vi "3.11-Threshold Lidar Data.vi"(2 "Angle Array":dbl[](array[numeric]), 3 "Magnitude Array":dbl[](array[numeric])) -> (0 "Y (mm)":dbl[](array[numeric]), 1 "X (mm)":dbl[](array[numeric]))   [LabVIEW 2010]
uses:
  3.0-Global.vi
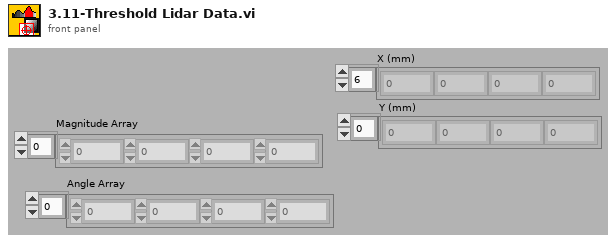
[diagram p1: front panel]
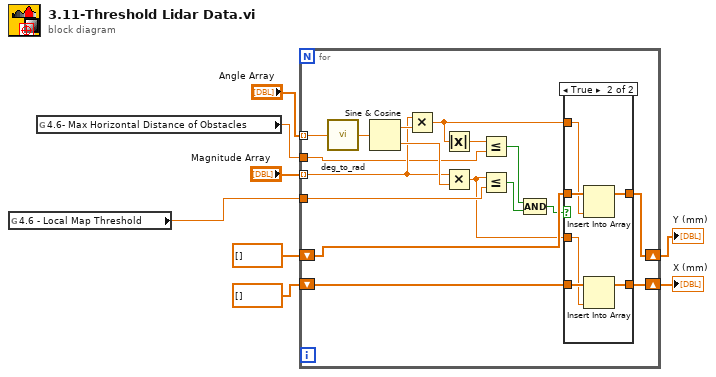
[diagram p0: block diagram]
diagram:
  n1 = global read "3.0-Global.vi" "4.6 - Local Map Threshold"() -> (w1:dbl)
  n2 = global read "3.0-Global.vi" "4.6- Max Horizontal Distance of Obstacles"() -> (w2:dbl)
  n3 = for {
    tunnel: "Magnitude Array" -> [w16] mode=indexing
    shift-right: [w25] -> w6
    shift-left: dbl[] [] -> [w23]
    shift-right: [w24] -> w5
    shift-left: dbl[] [] -> [w22]
    tunnel: "Angle Array" -> [w20] mode=indexing
    tunnel: w1 -> [w18]
    tunnel: w2 -> [w10]
    n4 = call "deg_to_rad.vi"("Degrees"=w20) -> ("Radians"=w21:dbl)
    n5 = Sine & Cosine(0:w21) -> (1:w19:dbl, 2:w17:dbl)
    n6 = Multiply(x=w16, y=w19) -> (x*y=w15:dbl)
    n7 = Absolute Value(x=w15) -> (abs(x)=w14:dbl)
    n8 = Multiply(x=w16, y=w17) -> (x*y=w9:dbl)
    n9 = Less Or Equal?(x=w14, y=w10) -> (x <= y?=w13:bool)
    n10 = Less Or Equal?(x=w9, y=w18) -> (x <= y?=w12:bool)
    n11 = Compound Arithmetic op=AND(w13, w12) -> (w11:bool)
    n12 = case shown="True" w11 {
      tunnel: [w27 w33] -> w25
      tunnel: [w26 w32] -> w24
      tunnel: w23 -> [w27 w31]
      tunnel: w22 -> [w26 w30]
      tunnel: w15 -> [_ w29]
      tunnel: w9 -> [_ w28]
      frame False {
      }
      frame True {
        n13 = Insert Into Array(array=w30, new element=w29) -> (w32:dbl[])  [unwired: 1 in]
        n14 = Insert Into Array(array=w31, new element=w28) -> (w33:dbl[])  [unwired: 1 in]
      }
    }
  }
  "X (mm)" <- w6
  "Y (mm)" <- w5
